vi "Reserve Sessions - NPin.vi"(6 "timeout (ms)":i32, 8 "error in":errorcluster, 10 "pin or relay names":string[](array[string]), 11 "measurement context in":refnum<class "Measure Call Context.lvclass">) -> (0 "error out":errorcluster, 2 "session reservation out":refnum<class "Session Reservation.lvclass">, 3 "measurement context out":refnum<class "Measure Call Context.lvclass">)   [LabVIEW 2020, in "Plug-In SDK Measurement.lvlib" / "Measure Call Context.lvclass"]
doc: "Reserves session(s) based on the provided pin information."
uses:
  Measure Call Context.lvclass
  Clients/Session Management V1/Session Reservation/Session Reservation.lvclass
  C:/dev/measurementlink-labview/Source/Runtime/Clients/Session Management V1/IReservation Observer/IReservation Observer.lvclass
  Helpers/Error Strings Global Internal.vi
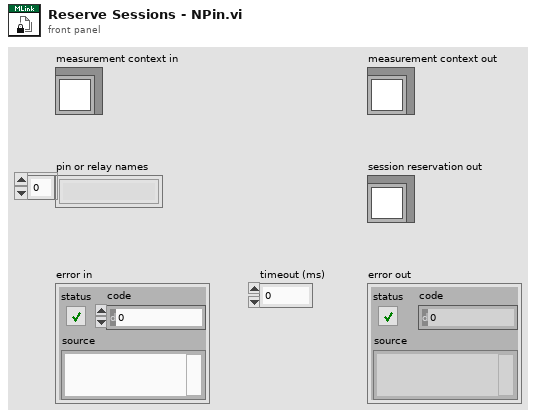
[diagram p1: front panel]
types:
  T1 = typedef "Plug-In SDK Measurement.lvlib/Pin Map Context.ctl" = cluster{"pin map id":string, "sites":i32[]}
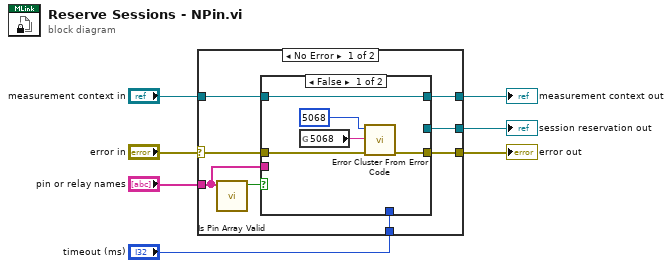
[diagram p0: block diagram]
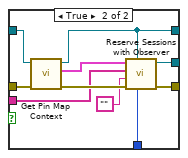
[diagram p2: hidden frame]
diagram:
  n1 = case shown="No Error" "error in" {
    selector: "error in" -> [w12 w31]
    tunnel: [w15 w31] -> w7
    tunnel: [w14 _] -> w6
    tunnel: "timeout (ms)" -> [w11 _]
    tunnel: "pin or relay names" -> [w8 _]
    tunnel: [w10 w32] -> w3
    tunnel: "measurement context in" -> [w13 w32]
    frame No Error {
      n2 = call "Is Pin Array Valid.vi"("pin or relay names"=w8) -> ("valid"=w9:bool)  [unwired: 10 in]
      n3 = case shown="False" w9 {
        tunnel: [w18 w30] -> w15
        tunnel: [_ w29] -> w14
        tunnel: w8 -> [_ w26]
        tunnel: w13 -> [w17 w25]
        tunnel: w12 -> [w19 w24]
        tunnel: w11 -> [_ w22]
        tunnel: [w17 w21] -> w10
        frame False {
          n4 = global read "Error Strings Global Internal.vi" "5068"() -> (w20:string)
          n5 = call <vilib>:"Error Cluster From Error Code.vi"("error in (no error)"=w19, "error message (\"\")"=w20, "error code (0)"=5068) -> ("error out"=w18:errorcluster)  [unwired: 6 in]
        }
        frame True {
          n6 = call-dynamic "Get Pin Map Context.vi"("error in"=w24, "measure call context in"=w25) -> ("error out"=w27:errorcluster, "pin map context"=w28:T1, "measure call context out"=w21:refnum<class "Measure Call Context.lvclass">)  [unwired: 7 in]
          n7 = call "Reserve Sessions with Observer.vi"("timeout (ms)"=w22, "reservation observer"=w21, "error in"=w27, "instrument type id"="" ("instrument_type_id"), "pin or relay names"=w26, "pin map context"=w28) -> ("error out"=w30:errorcluster, "session reservation out"=w29:refnum<class "Session Reservation.lvclass">)  [unwired: 4 in]
        }
      }
    }
    frame Error {
    }
  }
  "error out" <- w7
  "session reservation out" <- w6
  "measurement context out" <- w3
